vi "WT500 Configure Array Locations.vi"(8 "error in (no error)":errorcluster, 10 "Display Format":u16(ring) items=["Numeric", "Wave", "Bar", "Vector", "Trend"], 11 "VISA Refnum in":refnum<visa-resource-name>) -> (0 "error out":errorcluster, 1 "Array of Measurements":u16[](array[numeric]), 2 "Array Locations":u16[](array[numeric]), 3 "VISA Refnum out":refnum<visa-resource-name>)   [LabVIEW 2018]
uses:
  LLBs/ykwt500.llb/YKWT500 Configure Numeric Item (Set).vi
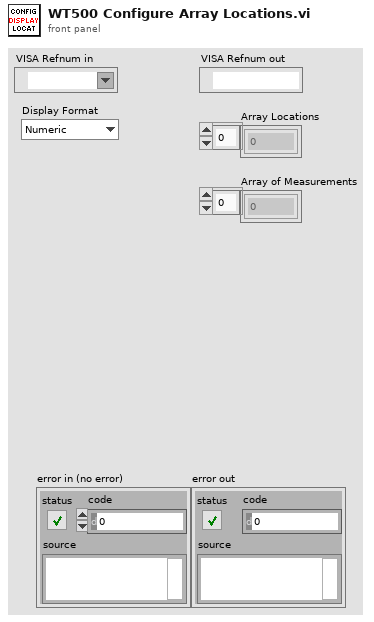
[diagram p1: front panel]
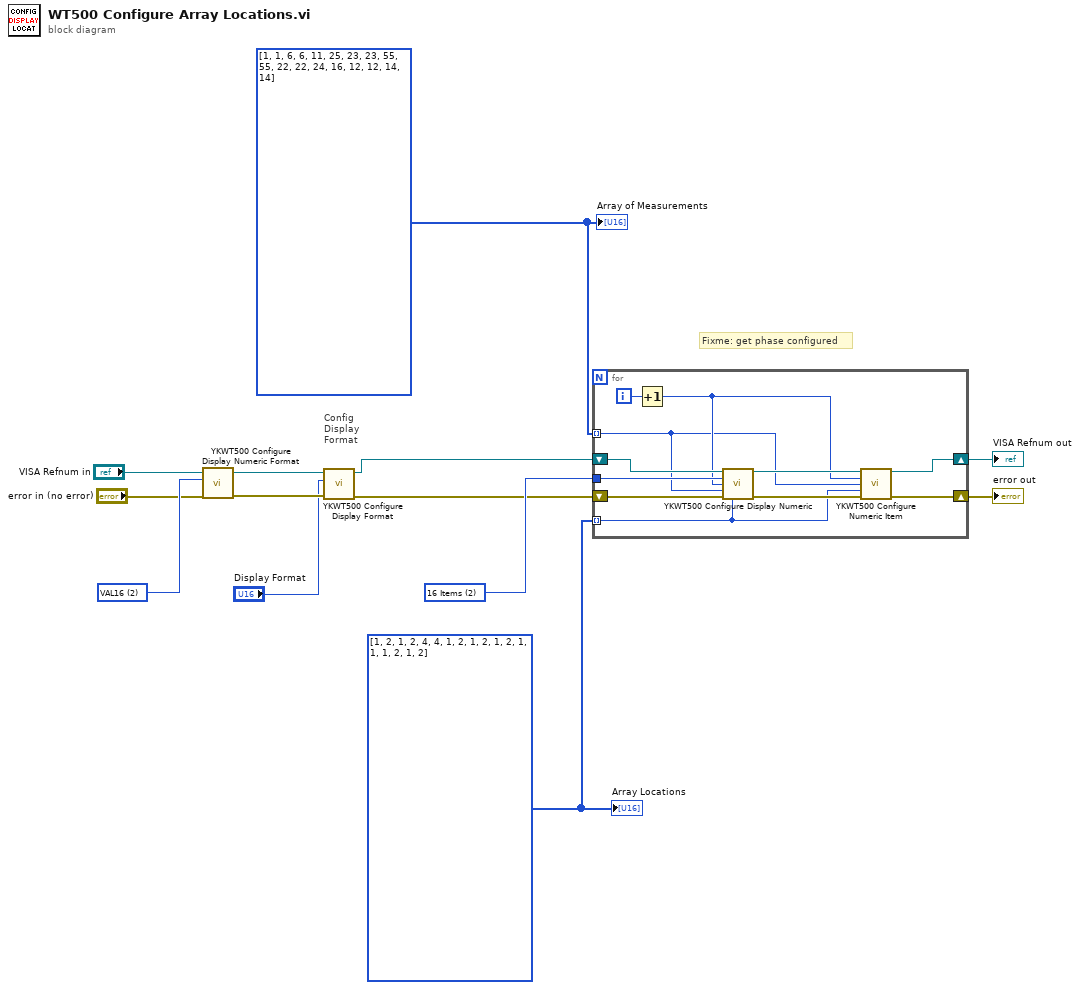
[diagram p0: block diagram]
diagram:
  w5 = u16 2 items=["VAL4", "VAL8", "VAL16", "MATRIX", "ALL"] ("Display Format (0: Numeric)")
  w9 = u16[] [1, 2, 1, 2, 4, 4, 1, 2, 1, 2, 1, 2, 1, 1, 1, 2, 1, 2] items=["NONE", "Element 1", "Element 2", "Element 3", "Sigma"]
  w10 = u16[] [1, 1, 6, 6, 11, 25, 23, 23, 55, 55, 22, 22, 24, 16, 12, 12, 14, 14] items=["None", "Urms", "Umn", "Udc", "Urmn", "Uac", "Irms", "Imn", "Idc", "Irmn", "Iac", "P", "S", "Q", "Lambda", "Phi", "Freq U", "Freq I", "U +peak", "U -peak", "I +peak", "I -peak", "Cf U", "Cf I", "Time", "Wp", "Wp+", "Wp-", "q", "q+", "q-", "WS", "WQ", "Eta 1", "Eta 2", "F1", "F2", "F3", "F4", "F5", "F6", "F7", "F8", "U(k)", "I(k)", "P(k)", "S(k)", "Q(k)", "Lambda(k)", "Phi(k)", "Phi U(k)", "Phi I(k)", "Uhdf(k)", "Ihdf(k)", "Phdf(k)", "Uthd", "Ithd", "Pthd", "Phi Ui-Uj", "Phi Ui-Uk", "Phi Ui-Ii", "Phi Ui-Ij", "Phi Ui-Ik", "Delta 1", "Delta 2", "Delta 3", "Delta 4"] ("Array of Measurements")
  w11 = u16 2 items=["4 Items", "8 Items", "16 Items", "Matrix"] ("Numeric Format (0: 4 Items)")
  # "Config\nDisplay\nFormat"
  # "Fixme: get phase configured"
  n1 = call "YKWT500 Configure Display Numeric Format.vi"("error in (no error)"="error in (no error)", "Numeric Format (0: 4 Items)"=w5, "VISA resource name"="VISA Refnum in") -> ("error out"=w7:errorcluster, "VISA resource name out"=w8:refnum<visa-resource-name>)  [unwired: 7 in]
  n2 = call "YKWT500 Configure Display Format.vi"("error in (no error)"=w7, "Display Format (0: Numeric)"="Display Format", "VISA resource name"=w8) -> ("error out"=w2:errorcluster, "VISA resource name out"=w1:refnum<visa-resource-name>)  [unwired: 7 in]
  n3 = for {
    shift-right: [w18] -> w12
    shift-left: w1 -> [w24]
    shift-right: [w19] -> w13
    shift-left: w2 -> [w23]
    tunnel: w11 -> [w21]
    tunnel: w9 -> [w16] mode=indexing
    tunnel: w10 -> [w14] mode=indexing
    i -> [w22]
    n4 = Increment(x=w22) -> (x+1=w15:i32)
    n5 = call "YKWT500 Configure Display Numeric.vi"("VISA resource name"=w24, "Numeric Format (0: 4 Items)"=w21, "Numeric Item Number (1)"=w15, "Numeric Function (0: None)"=w14, "error in (no error)"=w23, "Element (1: Element 1)"=w16) -> ("VISA resource name out"=w17:refnum<visa-resource-name>, "error out"=w20:errorcluster)  [unwired: 8 in]
    n6 = call-poly "YKWT500 Configure Numeric Item.vi"("VISA resource name"=w17, "Numeric Item Number (1)"=w15, "Numeric Function (0: None)"=w14, "Element (1: Element 1)"=w16, "error in (no error)"=w20) -> ("VISA resource name out"=w18:refnum<visa-resource-name>, "error out"=w19:errorcluster)  [unwired: 9 in]
  }
  "error out" <- w13
  "VISA Refnum out" <- w12
  "Array of Measurements" <- w10
  "Array Locations" <- w9
